vi "SP Check for Equality.vi"(3 "n2":dbl format="%0.17f", 4 "n1":dbl format="%0.17f") -> (0 "measured precision":i32, 1 "equal?":bool)   [LabVIEW 2011]
doc: "Check two floating point numbers for equality. Equality is defined as equal to 6 orders of magnitude. When comparing two numbers which are supposed to be zero, if one is zero, the other must be 1E-6 or less to get equality. If both are non-zero, they are compared as usual. This may cause errors for two numbers supposed to be zero, but with round-off error so they are not zero."
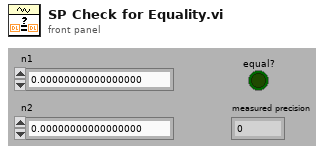
[diagram p1: front panel]
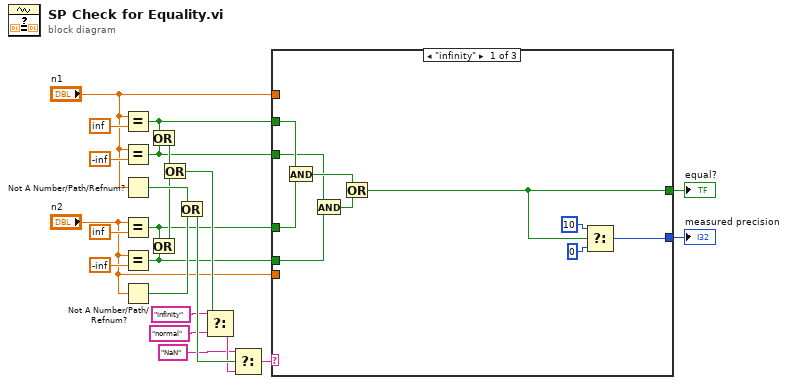
[diagram p0: block diagram]
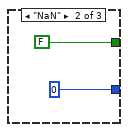
[diagram p2: hidden frame]
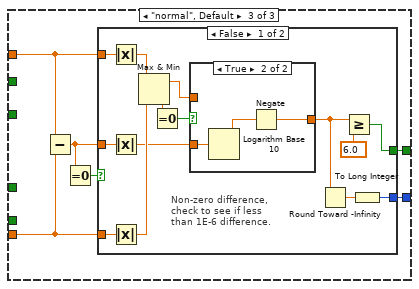
[diagram p3: hidden frame]
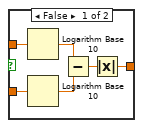
[diagram p4: hidden frame]
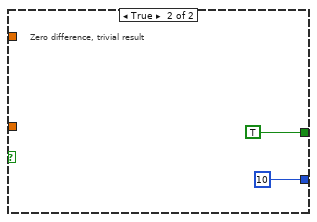
[diagram p5: hidden frame]
diagram:
  n1 = Equal?(x="n1", y=inf) -> (x = y?=w7:bool)
  n2 = Equal?(x="n1", y=-inf) -> (x = y?=w8:bool)
  n3 = Not A Number/Path/Refnum?(number/path/refnum="n1") -> (NaN/Path/Refnum?=w19:bool)
  n4 = Equal?(x="n2", y=inf) -> (x = y?=w6:bool)
  n5 = Equal?(x="n2", y=-inf) -> (x = y?=w5:bool)
  n6 = Not A Number/Path/Refnum?(number/path/refnum="n2") -> (NaN/Path/Refnum?=w18:bool)
  n7 = Or(x=w7, y=w8) -> (x .or. y?=w17:bool)
  n8 = Or(x=w6, y=w5) -> (x .or. y?=w16:bool)
  n9 = Or(x=w17, y=w16) -> (x .or. y?=w15:bool)
  n10 = Or(x=w19, y=w18) -> (x .or. y?=w14:bool)
  n11 = Select(t="infinity", s=w15, f="normal") -> (s? t:f=w13:string)
  n12 = Select(t="NaN", s=w14, f=w13) -> (s? t:f=w9:string)
  n13 = case shown="\"infinity\"" w9 {
    tunnel: [w26 FALSE w37] -> w3
    tunnel: [w27 0 w36] -> w2
    tunnel: w8 -> [w28 _ _]
    tunnel: w7 -> [w33 _ _]
    tunnel: w6 -> [w32 _ _]
    tunnel: w5 -> [w29 _ _]
    tunnel: "n1" -> [_ _ w39]
    tunnel: "n2" -> [_ _ w38]
    frame "infinity" {
      n14 = And(x=w33, y=w32) -> (x .and. y?=w31:bool)
      n15 = And(x=w28, y=w29) -> (x .and. y?=w30:bool)
      n16 = Or(x=w31, y=w30) -> (x .or. y?=w26:bool)
      n17 = Select(t=10, s=w26, f=0) -> (s? t:f=w27:i32)
    }
    frame "NaN" {
    }
    frame "normal", Default {
      n18 = Subtract(x=w39, y=w38) -> (x-y=w40:dbl)
      n19 = Equal To 0?(x=w40) -> (x = 0?=w41:bool)
      n20 = case shown="False" w41 {
        tunnel: w40 -> [w55 _]
        tunnel: w39 -> [w49 _]
        tunnel: w38 -> [w48 _]
        tunnel: [w51 TRUE] -> w37
        tunnel: [w50 10] -> w36
        frame False {
          # "Non-zero difference,\ncheck to see if less\nthan 1E-6 difference."
          n21 = Absolute Value(x=w49) -> (abs(x)=w47:dbl)
          n22 = Absolute Value(x=w55) -> (abs(x)=w44:dbl)
          n23 = Absolute Value(x=w48) -> (abs(x)=w46:dbl)
          n24 = Max & Min(x=w47, y=w46) -> (max(x,y)=w42:dbl, min(x,y)=w43:dbl)
          n25 = Equal To 0?(x=w43) -> (x = 0?=w45:bool)
          n26 = case shown="True" w45 {
            tunnel: [w56 w62] -> w52
            tunnel: w42 -> [w58 _]
            tunnel: w44 -> [w57 w64]
            frame False {
              n27 = Logarithm Base 10(1:w58) -> (0:w61:dbl)
              n28 = Logarithm Base 10(1:w57) -> (0:w60:dbl)
              n29 = Subtract(x=w61, y=w60) -> (x-y=w59:dbl)
              n30 = Absolute Value(x=w59) -> (abs(x)=w56:dbl)
            }
            frame True {
              n31 = Logarithm Base 10(1:w64) -> (0:w63:dbl)
              n32 = Negate(x=w63) -> (-x=w62:dbl)
            }
          }
          n33 = Round Toward -Infinity(1:w52) -> (0:w53:dbl)
          n34 = Greater Or Equal?(x=w52, y=6.0) -> (x >= y?=w51:bool)
          n35 = To Long Integer(number=w53) -> (32bit integer=w50:i32)
        }
        frame True {
          # "Zero difference, trivial result"
        }
      }
    }
  }
  "measured precision" <- w2
  "equal?" <- w3
